vi "Configure CAN.vi"(0 "Source (0:Channel1)":u16(ring) items=["Channel 1", "Channel 2", "Channel 3", "Channel 4"], 5 "Signal Type (0:Differential)":u16(ring) items=["Differential", "CAN + H", "CAN - L", "TX", "RX"], 7 "Data Threshold (0.0V)":dbl, 9 "Nominal Bit Rate (1MB)":dbl=1000000.0, 11 "Trigger Condition (0:Start)":u16(ring) items=["Start", "Frame", "Identifier", "Data", "Identifier and Data", "EOF", "Missing ack"], 12 "CAN Format (0:Standard)":u16(ring) items=["Standard", "Extended"]) -> (10 "Output String":string)   [LabVIEW 2015, in "Tektronix 7000 Series.lvlib"]
doc: "Configure the common settings for the CAN trigger."
uses:
  <instrlib>/Tektronix 7000 Series/Tektronix 7000 Series.lvlib
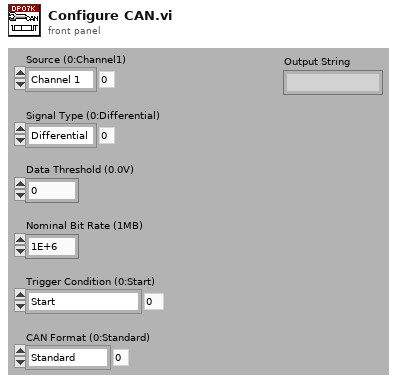
[diagram p1: front panel]
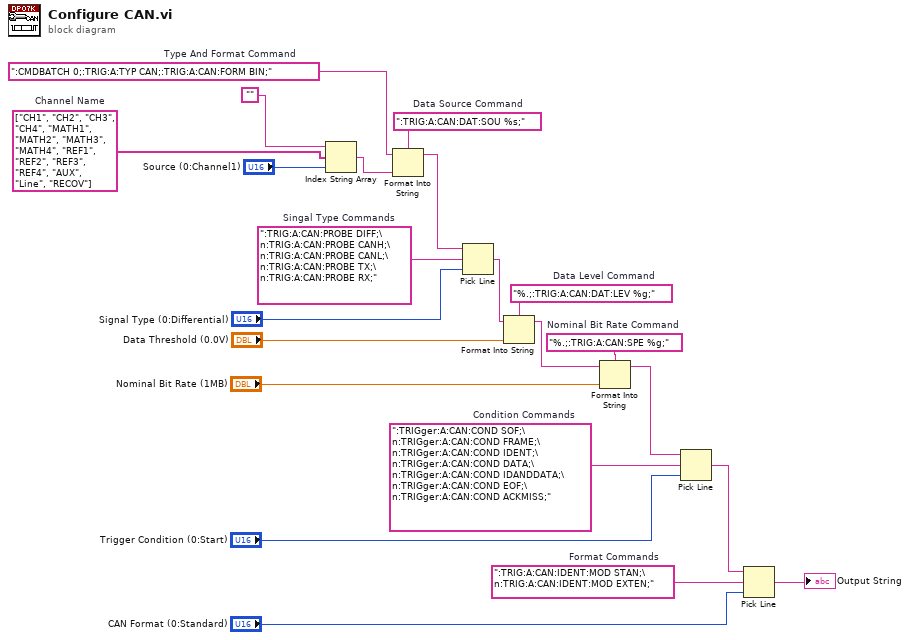
[diagram p0: block diagram]
diagram:
  w21 = ":TRIG:A:CAN:IDENT:MOD STAN;\n:TRIG:A:CAN:IDENT:MOD EXTEN;"  # Format Commands
  w19 = ":TRIGger:A:CAN:COND SOF;\n:TRIGger:A:CAN:COND FRAME;\n:TRIGger:A:CAN:COND IDENT;\n:TRIGger:A:CAN:COND DATA;\n:TRIGger:A:CAN:COND IDANDDATA;\n:TRIGger:A:CAN:COND EOF;\n:TRIGger:A:CAN:COND ACKMISS;"  # Condition Commands
  w16 = "%.;:TRIG:A:CAN:SPE %g;"  # Nominal Bit Rate Command
  w13 = "%.;:TRIG:A:CAN:DAT:LEV %g;"  # Data Level Command
  w11 = ":TRIG:A:CAN:PROBE DIFF;\n:TRIG:A:CAN:PROBE CANH;\n:TRIG:A:CAN:PROBE CANL;\n:TRIG:A:CAN:PROBE TX;\n:TRIG:A:CAN:PROBE RX;"  # Singal Type Commands
  w9 = ":TRIG:A:CAN:DAT:SOU %s;"  # Data Source Command
  w8 = ":CMDBATCH 0;:TRIG:A:TYP CAN;:TRIG:A:CAN:FORM BIN;"  # Type And Format Command
  w6 = string[] ["CH1", "CH2", "CH3", "CH4", "MATH1", "MATH2", "MATH3", "MATH4", "REF1", "REF2", "REF3", "REF4", "AUX", "Line", "RECOV"]  # Channel Name
  n1 = Index String Array(1:"Source (0:Channel1)", 2:w6, 3:"" ("Empty String Constant")) -> (0:w7:string)
  n2 = Format Into String(format string=w9, initial string=w8, w7) -> (resulting string=w10:string)  [unwired: 1 in, 1 out]
  n3 = Pick Line(string ("")=w10, multi-line string=w11, line index="Signal Type (0:Differential)") -> (output string=w12:string)
  n4 = Format Into String(format string=w13, initial string=w12, "Data Threshold (0.0V)") -> (resulting string=w15:string)  [unwired: 1 in, 1 out]
  n5 = Format Into String(format string=w16, initial string=w15, "Nominal Bit Rate (1MB)") -> (resulting string=w18:string)  [unwired: 1 in, 1 out]
  n6 = Pick Line(string ("")=w18, multi-line string=w19, line index="Trigger Condition (0:Start)") -> (output string=w20:string)
  n7 = Pick Line(string ("")=w20, multi-line string=w21, line index="CAN Format (0:Standard)") -> (output string=→"Output String":string)
